vi "Rawdata.vi"(1 "input rawdata":T1, 2 "set":bool) -> (0 "output rawdata":T1)   [LabVIEW 2009]
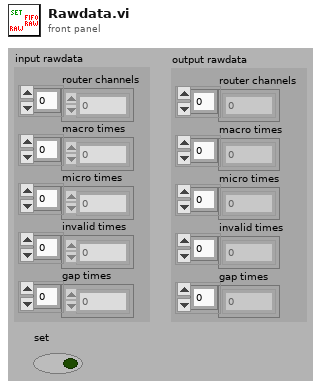
[diagram p1: front panel]
types:
  T1 = cluster{"router channels":u8[], "macro times":dbl[], "micro times":u16[], "invalid times":u32[], "gap times":u32[]}
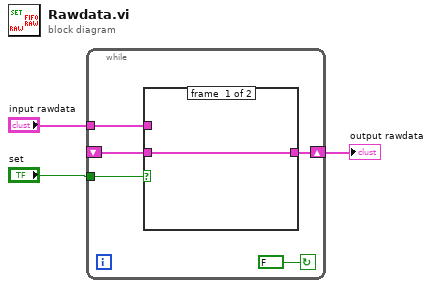
[diagram p0: block diagram]
diagram:
  n1 = while {
    shift-right: [w6] -> w3
    shift-left: _ -> [w4]
    tunnel: "set" -> [w7]
    tunnel: "input rawdata" -> [w5]
    stop <- FALSE continue-if-true
    n2 = case shown="False" w7 {
      tunnel: [w9 w10] -> w6
      tunnel: w5 -> [_ w10]
      tunnel: w4 -> [w9 _]
      frame #0 {
      }
      frame #1 {
      }
    }
  }
  "output rawdata" <- w3
